vi "Buy.vi"(8 "error in (no error)":errorcluster, 10 "Producto":string[](array[string]), 11 "UI Actor in":refnum<class "UI Actor.lvclass">) -> (0 "error out":errorcluster, 3 "UI Actor out":refnum<class "UI Actor.lvclass">)   [LabVIEW 2020, in "UI Actor.lvlib" / "UI Actor.lvclass"]
uses:
  UI Actor.lvclass
  C:/Program Files (x86)/National Instruments/LabVIEW 2020/vi.lib/ActorFramework/Actor/Actor.lvclass
  <vilib>/ActorFramework/Actor/Actor.lvclass/Actor.ctl
  <vilib>/ActorFramework/Message Enqueuer/Message Enqueuer.lvclass/Message Enqueuer.ctl
  UI Actor.lvclass/UI Actor.ctl
  UI Actor Messages/Actualiza MSG Msg/Actualiza MSG Msg.lvclass/Actualiza MSG Msg.ctl
  UI Actor Messages/Credit Purchase Msg/Credit Purchase Msg.lvclass/Credit Purchase Msg.ctl
  <vilib>/ActorFramework/Message Enqueuer/Init from Existing Queue.vi
  <vilib>/ActorFramework/Message Enqueuer/Enqueue.vi
  UI Actor Messages/Actualiza MSG Msg/Actualiza MSG Msg.lvclass
  C:/Program Files (x86)/National Instruments/LabVIEW 2020/vi.lib/ActorFramework/Message/Message.lvclass
  Cafe Messages/init Msg/init Msg.lvclass
  Coca Messages/Init Msg/Init Msg.lvclass
  UI Actor Messages/Credit Purchase Msg/Credit Purchase Msg.lvclass
  <vilib>/ActorFramework/Message Priority Queue/Priority Enqueue.vi
  <vilib>/ActorFramework/Message Enqueuer/Message Enqueuer.lvclass
  <vilib>/ActorFramework/Actor/Actor.lvclass
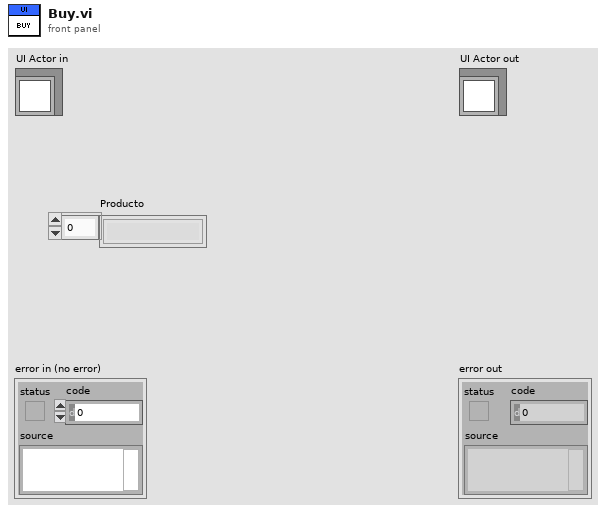
[diagram p1: front panel]
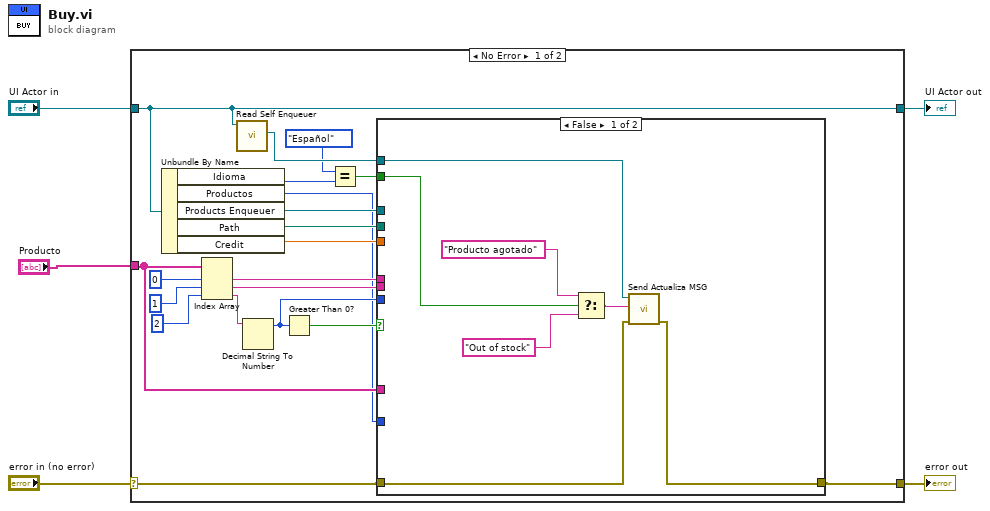
[diagram p0: block diagram]
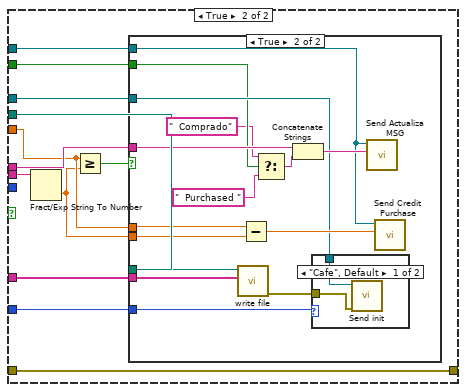
[diagram p2: hidden frame]
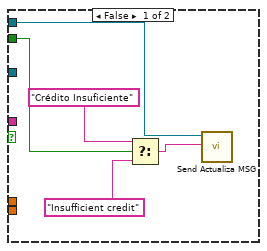
[diagram p3: hidden frame]
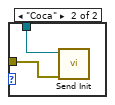
[diagram p4: hidden frame]
diagram:
  n1 = case shown="No Error" "error in (no error)" {
    selector: "error in (no error)" -> [w17 w70]
    tunnel: [w16 w70] -> w4
    tunnel: [w14 w69] -> w2
    tunnel: "UI Actor in" -> [w14 w69]
    tunnel: "Producto" -> [w11 _]
    frame No Error {
      n2 = Unbundle By Name(w14) -> ("Idioma"=w8:enum16{"Español", "Ingles"}, "Productos"=w9:enum16{"Cafe", "Coca"}, "Products Enqueuer"=w10:refnum<class "Message Enqueuer.lvclass">, "Path"=w12:path, "Credit"=w18:dbl)
      n3 = Index Array(array=w11, index #1=0 ("index"), index #2=1 ("index"), index #3=2 ("index")) -> (element #1=w21:string, element #2=w20:string, element #3=w19:string)
      n4 = call <vilib>:"Read Self Enqueuer.vi"("Actor"=w14) -> ("Self Enqueuer"=w13:refnum<class "Message Enqueuer.lvclass">)  [unwired: 10 in]
      n5 = Decimal String To Number(string=w19) -> (number=w15:i32)  [unwired: 2 in, 1 out]
      n6 = Greater Than 0?(x=w15) -> (x > 0?=w22:bool)
      n7 = Equal?(x=enum16{"Español", "Ingles"}."Español" ("y"), y=w8) -> (x = y?=w7:bool)
      n8 = case shown="False" w22 {
        tunnel: w21 -> [_ w40]
        tunnel: w20 -> [_ w43]
        tunnel: w18 -> [_ w39]
        tunnel: w13 -> [w32 w41]
        tunnel: w17 -> [w31 w44]
        tunnel: [w30 w44] -> w16
        tunnel: w15 -> [_ _]
        tunnel: w12 -> [_ w37]
        tunnel: w11 -> [_ w36]
        tunnel: w10 -> [_ w35]
        tunnel: w9 -> [_ w34]
        tunnel: w7 -> [w27 w33]
        frame False {
          n9 = Select(t="Producto agotado" ("MSG"), s=w27, f="Out of stock" ("t")) -> (s? t:f=w28:string)
          n10 = call "Send Actualiza MSG.vi"("error in (no error)"=w31, "MSG"=w28, "Message Enqueuer"=w32) -> ("error out"=w30:errorcluster)  [unwired: 7 in, 1 out]
        }
        frame True {
          n11 = Fract/Exp String To Number(string=w43) -> (number=w38:dbl)  [unwired: 3 in, 1 out]
          n12 = Greater Or Equal?(x=w39, y=w38) -> (x >= y?=w42:bool)
          n13 = case shown="True" w42 {
            tunnel: w41 -> [w49 w60]
            tunnel: w40 -> [_ w63]
            tunnel: w39 -> [_ w62]
            tunnel: w38 -> [_ w61]
            tunnel: w37 -> [_ w58]
            tunnel: w36 -> [_ w57]
            tunnel: w35 -> [_ w56]
            tunnel: w34 -> [_ w54]
            tunnel: w33 -> [w46 w53]
            frame False {
              n14 = Select(t="Crédito Insuficiente" ("MSG"), s=w46, f="Insufficient credit" ("t")) -> (s? t:f=w48:string)
              n15 = call "Send Actualiza MSG.vi"("MSG"=w48, "Message Enqueuer"=w49) -> ()  [unwired: 8 in, 2 out]
            }
            frame True {
              n16 = call "write file.vi"("Item Names"=w57, "configuration file path"=w58) -> ("error out"=w55:errorcluster)  [unwired: 9 in]
              n17 = Subtract(x=w62, y=w61) -> (x-y=w59:dbl)
              n18 = Select(t="  Comprado" ("MSG"), s=w53, f="  Purchased ") -> (s? t:f=w51:string)
              n19 = Concatenate Strings(w63, w51) -> (w64:string)
              n20 = case shown="\"Cafe\", Default" w54 {
                tunnel: w56 -> [w66 w68]
                tunnel: w55 -> [w65 w67]
                frame "Cafe", Default {
                  n21 = call "Send init.vi"("error in (no error)"=w65, "Message Enqueuer"=w66) -> ()  [unwired: 8 in, 2 out]
                }
                frame "Coca" {
                  n22 = call "Send Init.vi"("error in (no error)"=w67, "Message Enqueuer"=w68) -> ()  [unwired: 8 in, 2 out]
                }
              }
              n23 = call "Send Actualiza MSG.vi"("MSG"=w64, "Message Enqueuer"=w60) -> ()  [unwired: 8 in, 2 out]
              n24 = call "Send Credit Purchase.vi"("Credito"=w59, "Message Enqueuer"=w60) -> ()  [unwired: 8 in, 2 out]
            }
          }
        }
      }
    }
    frame Error {
    }
  }
  "error out" <- w4
  "UI Actor out" <- w2
